vi "PH_Image_Common.Overlay Ellipse.vi"(0 "Image":T1, 1 "Start Major Axis":cluster{"X":i32, "Y":i32}, 2 "End Major Axis":cluster{"X":i32, "Y":i32}, 3 "Start Minor Axis":cluster{"X":i32, "Y":i32}, 4 "End Minor Axis":cluster{"X":i32, "Y":i32}, 5 "error in (no error)":errorcluster, 8 "COG Ellipse":cluster{"X":i32, "Y":i32}, 9 "Color (red)":u32(colorbox)=16711680) -> (14 "Image Out":T1, 19 "error out":errorcluster)   [LabVIEW 2014, in "PH_Image_Common.lvlib"]
doc: "This VI overlays an ellipse to an image"
uses:
  <vilib>/vision/Image Controls.llb/IMAQ Image.ctl
  PH_Image_Common.lvlib
panel:
  in  "Lines":i32=60 min=2 max=400 step=1
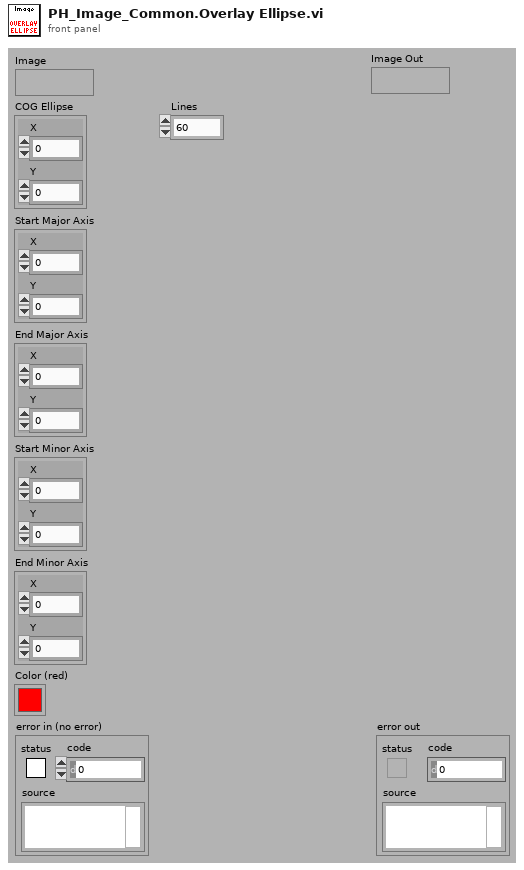
[diagram p1: front panel]
types:
  T1 = typedef "IMAQ Image.ctl" = refnum<image>
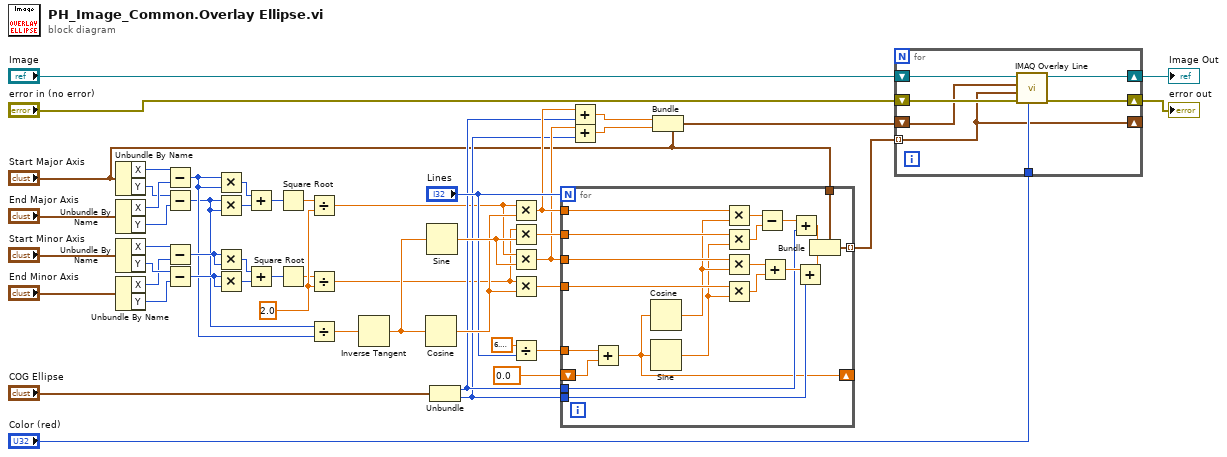
[diagram p0: block diagram]
diagram:
  w31 = 2.0 ("y")
  n1 = Unbundle By Name("Start Major Axis") -> ("X"=w48:i32, "Y"=w46:i32)
  n2 = Unbundle By Name("End Major Axis") -> ("X"=w47:i32, "Y"=w45:i32)
  n3 = Unbundle By Name("Start Minor Axis") -> ("X"=w33:i32, "Y"=w35:i32)
  n4 = Unbundle By Name("End Minor Axis") -> ("X"=w34:i32, "Y"=w36:i32)
  n5 = Subtract(x=w48, y=w47) -> (x-y=w25:i32)
  n6 = Subtract(x=w46, y=w45) -> (x-y=w24:i32)
  n7 = Subtract(x=w33, y=w34) -> (x-y=w37:i32)
  n8 = Subtract(x=w35, y=w36) -> (x-y=w38:i32)
  n9 = Multiply(x=w25, y=w25) -> (x*y=w43:i32)
  n10 = Multiply(x=w24, y=w24) -> (x*y=w44:i32)
  n11 = Multiply(x=w37, y=w37) -> (x*y=w40:i32)
  n12 = Multiply(x=w38, y=w38) -> (x*y=w39:i32)
  n13 = Add(x=w43, y=w44) -> (x+y=w42:i32)
  n14 = Add(x=w40, y=w39) -> (x+y=w41:i32)
  n15 = Square Root(x=w42) -> (sqrt(x)=w32:dbl)
  n16 = Square Root(x=w41) -> (sqrt(x)=w30:dbl)
  n17 = Divide(x=w32, y=w31) -> (x/y=w7:dbl)
  n18 = Divide(x=w30, y=w31) -> (x/y=w6:dbl)
  n19 = Divide(x=w24, y=w25) -> (x/y=w26:dbl)
  n20 = Inverse Tangent(1:w26) -> (0:w9:dbl)
  n21 = Cosine(x=w9) -> (cos(x)=w20:dbl)
  n22 = Sine(x=w9) -> (sin(x)=w21:dbl)
  n23 = Unbundle("COG Ellipse") -> ("X"=w13:i32, "Y"=w12:i32)
  n24 = Multiply(x=w7, y=w20) -> (x*y=w15:dbl)
  n25 = Multiply(x=w6, y=w21) -> (x*y=w23:dbl)
  n26 = Multiply(x=w7, y=w21) -> (x*y=w14:dbl)
  n27 = Multiply(x=w6, y=w20) -> (x*y=w22:dbl)
  n28 = Divide(x=6.283185307179586, y="Lines") -> (x/y=w17:dbl)
  n29 = for {
    N: "Lines" -> [_]
    tunnel: w17 -> [w71]
    tunnel: w15 -> [w70]
    tunnel: w23 -> [w69]
    tunnel: w14 -> [w68]
    tunnel: w22 -> [w67]
    shift-right: [w53] -> _
    shift-left: 0.0 -> [w72]
    tunnel: w13 -> [w58]
    tunnel: w12 -> [w57]
    tunnel: [w54] -> w1 mode=indexing
    tunnel: "Start Major Axis" -> [w52]
    n30 = Add(x=w71, y=w72) -> (x+y=w53:dbl)
    n31 = Cosine(x=w53) -> (cos(x)=w66:dbl)
    n32 = Sine(x=w53) -> (sin(x)=w65:dbl)
    n33 = Multiply(x=w70, y=w66) -> (x*y=w64:dbl)
    n34 = Multiply(x=w69, y=w65) -> (x*y=w63:dbl)
    n35 = Multiply(x=w68, y=w66) -> (x*y=w62:dbl)
    n36 = Multiply(x=w67, y=w65) -> (x*y=w61:dbl)
    n37 = Subtract(x=w64, y=w63) -> (x-y=w60:dbl)
    n38 = Add(x=w62, y=w61) -> (x+y=w59:dbl)
    n39 = Add(x=w60, y=w58) -> (x+y=w56:dbl)
    n40 = Add(x=w59, y=w57) -> (x+y=w55:dbl)
    n41 = Bundle(cluster=w52, "X"=w56, "Y"=w55) -> (w54:cluster{"X":i32, "Y":i32})
  }
  n42 = Add(x=w15, y=w13) -> (x+y=w11:dbl)
  n43 = Add(x=w14, y=w12) -> (x+y=w10:dbl)
  n44 = Bundle(cluster="Start Major Axis", "X"=w11, "Y"=w10) -> (w2:cluster{"X":i32, "Y":i32})
  n45 = for {
    tunnel: "Color (red)" -> [w75]
    shift-right: [w79] -> w51
    shift-left: "error in (no error)" -> [w77]
    shift-right: [w78] -> w50
    shift-left: "Image" -> [w76]
    tunnel: w1 -> [w73] mode=indexing
    shift-right: [w73] -> _
    shift-left: w2 -> [w74]
    n46 = call "IMAQ Overlay Line"("Color"=w75, "error in (no error)"=w77, "End Point"=w73, "Start Point"=w74, "Image"=w76) -> ("error out"=w79:errorcluster, "Image Out"=w78:T1)  [unwired: 5 in]
  }
  "error out" <- w51
  "Image Out" <- w50
